vi "Finalize Data.vi"(8 "error in (no error)":errorcluster, 11 "Core Transfers Configuration in":refnum<class "Core Transfers Configuration.lvclass">) -> (0 "error out":errorcluster, 1 "data version":T1, 2 "data":string, 3 "Core Transfers Configuration out":refnum<class "Core Transfers Configuration.lvclass">)   [LabVIEW 2017, in "DSF Core.lvlib" / "Core Transfers Configuration.lvclass"]
uses:
  Core Transfers Configuration.lvclass
  C:/Git/DSF/Core/Classes/Configuration/Configuration.lvclass
  Typedefs/DSF Version Info.ctl
  Core Transfers Configuration.lvclass/Core Transfers Configuration.ctl
  Configuration.lvclass
  DSF Core.lvlib
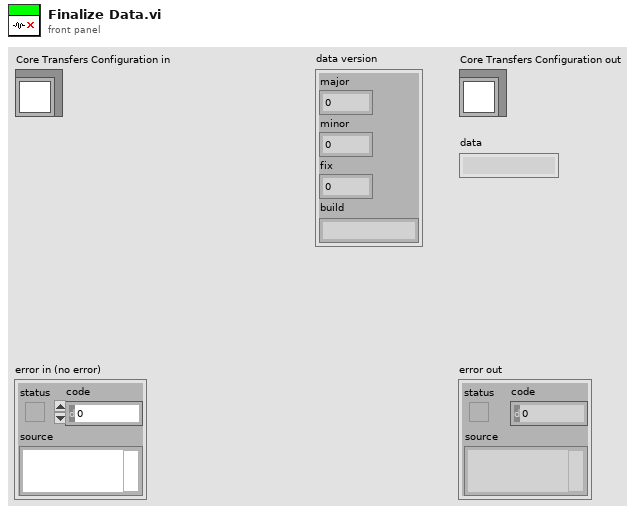
[diagram p1: front panel]
types:
  T1 = typedef "DSF Core.lvlib/DSF Version Info.ctl" = cluster{"major":i32, "minor":i32, "fix":i32, "build":string}
  T2 = typedef "DSF Core.lvlib/Core Transfers Configuration.lvclass/Configuration.ctl" = cluster{"name":string}
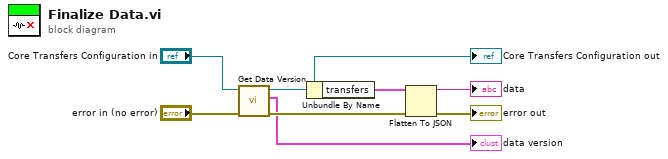
[diagram p0: block diagram]
diagram:
  n1 = call "Get Data Version.vi"("error in (no error)"="error in (no error)", "Configuration in"="Core Transfers Configuration in") -> ("error out"=w4:errorcluster, "data version"=→"data version":T1, "Configuration out"=w2:refnum<class "Core Transfers Configuration.lvclass">)  [unwired: 7 in]
  "Core Transfers Configuration out" <- w2
  n2 = Unbundle By Name(w2) -> ("transfers"=w8:T2[])
  n3 = Flatten To JSON(anything=w8, error in (no error)=w4) -> (JSON string=→"data":string, 11:→"error out":errorcluster)  [unwired: 1 in]
